vi "Load Default QD Object Shortcuts.vi"   [LabVIEW 2016]
uses:
  <resource>/dialog/lvconfig.llb/LV Config Read String.vi
  <resource>/dialog/lvconfig.llb/LV Config Write String.vi
panel:
  # "This VI loads the default set of QD object shortcuts for this language of LabVIEW into the INI file."
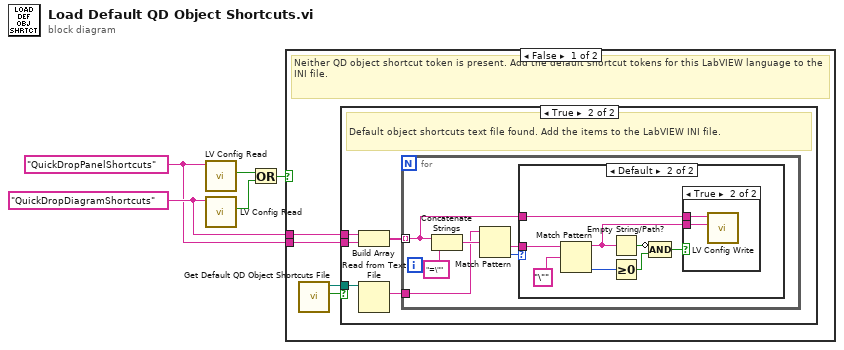
[diagram p0: block diagram]
diagram:
  w2 = "QuickDropDiagramShortcuts" ("Name")
  w1 = "QuickDropPanelShortcuts" ("Name")
  n1 = call-poly <resource>:"LV Config Read.vi"("key"=w1) -> ("found?"=w5:bool)  [unwired: 4 in, 2 out]
  n2 = call-poly <resource>:"LV Config Read.vi"("key"=w2) -> ("found?"=w4:bool)  [unwired: 4 in, 2 out]
  n3 = Or(x=w5, y=w4) -> (x .or. y?=w3:bool)
  n4 = case shown="False" w3 {
    tunnel: w2 -> [w9 _]
    tunnel: w1 -> [w8 _]
    frame False {
      # "Neither QD object shortcut token is present. Add the default shortcut tokens for this LabVIEW language to the INI file."
      n5 = call <resource>:"Get Default QD Object Shortcuts File.vi"() -> ("file exists"=w7:bool, "default shortcuts text file"=w6:path)  [unwired: 10 in]
      n6 = case shown="True" w7 {
        tunnel: w6 -> [_ w14]
        tunnel: w9 -> [_ w12]
        tunnel: w8 -> [_ w11]
        frame False {
          # "Default object shortcuts text file does not exist for this language. Do nothing."
        }
        frame True {
          # "Default object shortcuts text file found. Add the items to the LabVIEW INI file."
          n7 = Build Array(w12, w11) -> (w10:string[])
          n8 = Read from Text File(file (use dialog)=w14) -> (text=w13:string)  [unwired: 3 in, 3 out]
          n9 = for {
            tunnel: w13 -> [w16]
            tunnel: w10 -> [w18] mode=indexing
            n10 = Concatenate Strings(w18, "=\"") -> (w17:string)
            n11 = Match Pattern(string=w16, regular expression=w17) -> (after substring=w19:string, offset past match=w15:i32)  [unwired: 1 in, 2 out]
            n12 = case shown="Default" w15 {
              tunnel: w19 -> [_ w28]
              tunnel: w18 -> [_ w26]
              frame -1 {
              }
              frame Default {
                n13 = Match Pattern(string=w28, regular expression="\"") -> (before substring=w25:string, offset past match=w23:i32)  [unwired: 1 in, 2 out]
                n14 = Empty String/Path?(string/path=w25) -> (empty?=w24:bool)
                n15 = Greater Or Equal To 0?(x=w23) -> (x >= 0?=w22:bool)
                n16 = Compound Arithmetic op=AND(invert w24, w22) -> (w21:bool)
                n17 = case shown="True" w21 {
                  tunnel: w26 -> [_ w30]
                  tunnel: w25 -> [_ w29]
                  frame False {
                  }
                  frame True {
                    n18 = call-poly <resource>:"LV Config Write.vi"("value"=w29, "key"=w30) -> ()  [unwired: 5 in, 1 out]
                  }
                }
              }
            }
          }
        }
      }
    }
    frame True {
      # "One or both of the QD object shortcut tokens is already present, don't do anything with loading default shortcuts."
    }
  }
